vi "GAU2DArray.vi"(8 "Colums":i32=6, 11 "Rows":i32=3) -> (0 "2D Double Array":i32[][](array[numeric]), 3 "2D String Array":string[][](array[string]))   [LabVIEW 2023]
uses:
  <vilib>/numeric/Random Number (Range) DBL.vi
  <vilib>/numeric/Random Number (Range) U64.vi
  <vilib>/numeric/sub_Random U32.vi
panel:
  out "Repeated attempt":i32
  out "?":i32
  out "?":i32
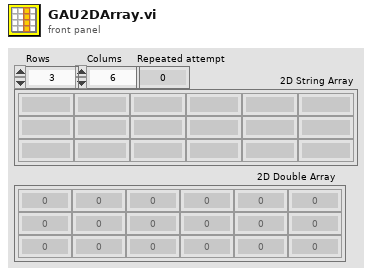
[diagram p1: front panel]
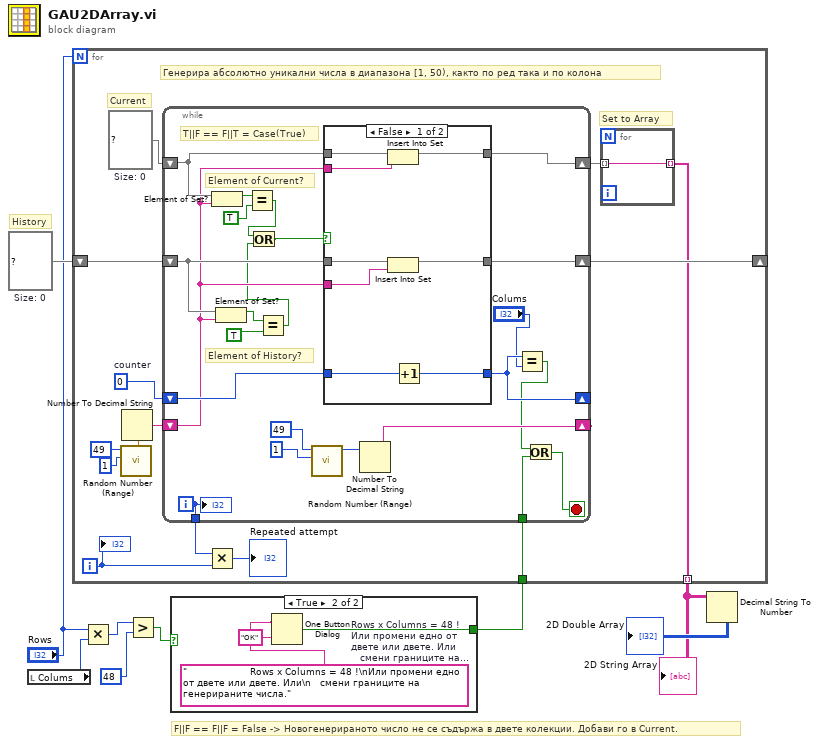
[diagram p0: block diagram]
diagram:
  w8 = set{string} {}  # Size: 0
  # "History"
  # "F||F == F||F = False -> Новогенерираното число не се съдържа в двете колекции. Добави го в Current."
  n1 = local read "Colums"() -> (w2:i32)
  n2 = Multiply(x="Rows", y=w2) -> (x*y=w1:i32)
  n3 = Greater?(x=w1, y=48) -> (0:w6:bool)
  n4 = case shown="True" w6 {
    selector: w6 -> [w10 _]
    tunnel: [w10 w11] -> w5
    frame False {
    }
    frame True {
      w13 = "                     Rows x Columns = 48 !\nИли промени едно от двете или двете. Или\n   смени границите на генерираните числа."  # Rows x Columns = 48 ! Или промени едно от двете или двете. Или    смени границите на генерираните числа.
      n5 = One Button Dialog(message=w13, button name ("OK")="ОК") -> (true=w11:bool)
    }
  }
  n6 = for {
    N: "Rows" -> [_]
    tunnel: [w14] -> w4 mode=indexing
    shift-right: [w20] -> _
    shift-left: w8 -> [w19]
    tunnel: w5 -> [w15]
    i -> [w17]
    w21 = set{string} {}  # Size: 0
    w23 = 0  # counter
    # "Current"
    # "Генерира абсолютно уникални числа в диапазона [1, 50), както по ред така и по колона"
    # "Set to Array"
    n7 = call-poly <vilib>:"Random Number (Range).vi"("lower bound (0)"=u64 1, "upper bound (100)"=u64 49) -> ("number"=w27:dbl)  [unwired: 9 in]
    n8 = Number To Decimal String(number=w27) -> (decimal integer string=w24:string)  [unwired: 1 in]
    n9 = while {
      shift-right: [w50] -> w22
      shift-left: w21 -> [w51]
      shift-right: [w43] -> _
      shift-left: w24 -> [w40]
      shift-right: [w48] -> _
      shift-left: w23 -> [w49]
      shift-right: [w42] -> w20
      shift-left: w19 -> [w41]
      tunnel: [w32] -> w18
      tunnel: w15 -> [w30]
      i -> [w32]
      stop <- w29 stop-if-true
      # "Element of Current?"
      # "Element of History?"
      # "T||F == F||T = Case(True)"
      n10 = Element of Set?(10:w40, 11:w51) -> (3:w37:bool)
      n11 = Element of Set?(10:w40, 11:w41) -> (3:w39:bool)
      n12 = Equal?(x=w37, y=TRUE) -> (x = y?=w34:bool)
      n13 = Equal?(x=w39, y=TRUE) -> (x = y?=w35:bool)
      n14 = Or(x=w34, y=w35) -> (x .or. y?=w33:bool)
      n15 = call-poly <vilib>:"Random Number (Range).vi"("lower bound (0)"=u64 1, "upper bound (100)"=u64 49) -> ("number"=w46:u64)  [unwired: 9 in]
      n16 = case shown="False" w33 {
        tunnel: w51 -> [w59 w62]
        tunnel: w40 -> [w57 _]
        tunnel: [w58 w62] -> w50
        tunnel: w49 -> [w55 w61]
        tunnel: [w56 w61] -> w48
        tunnel: [w52 w60] -> w42
        tunnel: w40 -> [w54 _]
        tunnel: w41 -> [w53 w60]
        frame False {
          n17 = Insert Into Set(10:w57, 11:w59) -> (3:w58:set{string})  [unwired: 1 out]
          n18 = Insert Into Set(10:w54, 11:w53) -> (3:w52:set{string})  [unwired: 1 out]
          n19 = Increment(x=w55) -> (x+1=w56:i32)
        }
        frame True {
        }
      }
      n20 = Number To Decimal String(number=w46) -> (decimal integer string=w43:string)  [unwired: 1 in]
      n21 = Equal?(x=w48, y="Colums") -> (x = y?=w31:bool)
      n22 = Or(x=w31, y=w30) -> (x .or. y?=w29:bool)
      "?" <- w32
    }
    n23 = Multiply(x=w18, y=w17) -> (x*y=→"Repeated attempt":i32)
    n24 = for {
      tunnel: [w28] -> w14 mode=indexing
      tunnel: w22 -> [w28] mode=indexing
    }
    "?" <- w17
  }
  "2D String Array" <- w4
  n25 = Decimal String To Number(string=w4) -> (number=→"2D Double Array":i32[][])  [unwired: 2 in, 1 out]
